vi "GetClassDependencies.vi"(0 "ClassReader in":refnum<class "ClassReader.lvclass">, 1 "DependencyVIs":T4[](array[typedef]), 2 "Attributes":T1[](array[typedef])=[{"name"="MyU8", "type"=enum."UINT8", "dimension"=0, "typeName"="", "typePath"=path "", "visibility"=enum."Protected"}, {"name"="MyStrArray", "type"=enum."STRING", "dimension"=1, "typeName"="", "typePath"=path "", "visibility"=enum."Protected"}], 5 "error in (no error)":errorcluster) -> (14 "ClassReader out":refnum<class "ClassReader.lvclass">, 15 "DependencyClassPaths":path[](array[path]), 16 "IsDependencyClassPathsAByValueClass":bool[](array[boolean]), 17 "CreateClassVIsCalled":path[](array[path]), 19 "error out":errorcluster)   [LabVIEW 2020, in "ClassReader.lvclass"]
uses:
  ClassReader.lvclass
  MethodDependencyType.ctl
  Common/ScriptingFunctions/SubVIs/Scripting_ViDependencyType.ctl
  Common/CommonVIs/CommonVIs_AttributeInfoType.ctl
  Common/CommonVIs/CommonVIs_AttributeDataType.ctl
  Common/CommonVIs/CommonVIs_VisibilityType.ctl
  ClassReader.lvclass/ClassReader.ctl
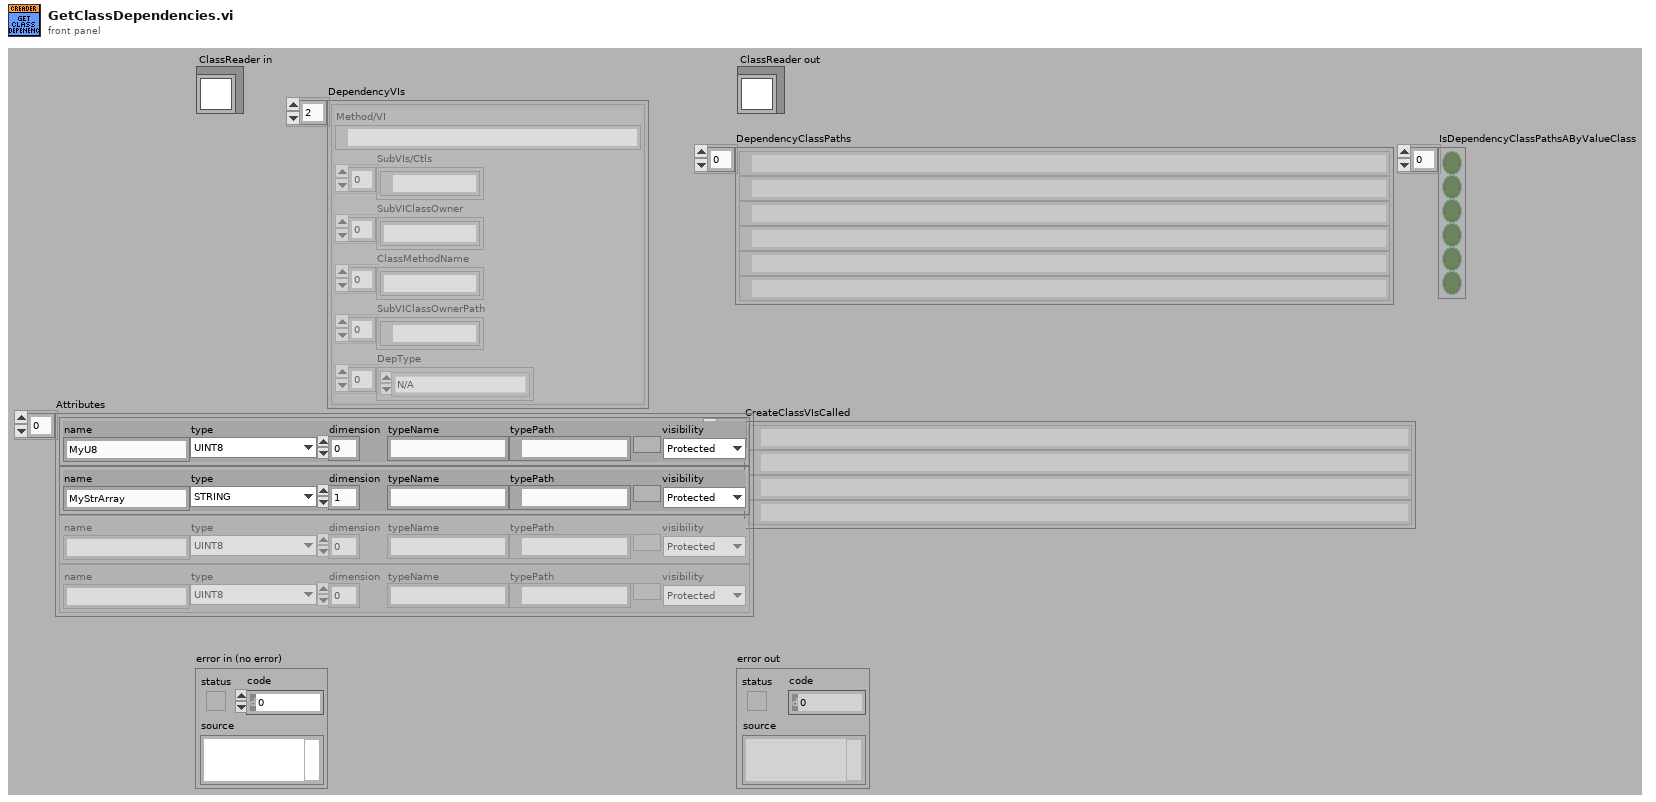
[diagram p1: front panel]
types:
  T1 = typedef "CommonVIs_AttributeInfoType.ctl" = cluster{"name":string, "type":T2, "dimension":i32, "typeName":string, "typePath":path, "visibility":T3}
  T2 = typedef "CommonVIs_AttributeDataType.ctl" = enum16{"UINT8", "INT8", "UINT16", "INT16", "UINT32", "INT32", "UINT64", "INT64", "SGL", "DBL", "EXT", "CSG", "CDB", "CXT", "TimeStamp", "STRING", "PATH", "BOOL", "ENUM", "RefNum", "VIRefNum", "LabVIEW Class", "Cluster", "Variant", "TypeDef", "Waveform", "LabVIEW Object", "Other", "void", "Set", "Map"}
  T3 = typedef "CommonVIs_VisibilityType.ctl" = enum16{"Public", "Private", "Protected"}
  T4 = typedef "ClassReader.lvclass/MethodDependencyType.ctl" = cluster{"Method/VI":path, "SubVIs/Ctls":path[], "SubVIClassOwner":string[], "ClassMethodName":string[], "SubVIClassOwnerPath":path[], "DepType":T5[]}
  T5 = typedef "Scripting_ViDependencyType.ctl" = enum16{"N/A", "Launches"}
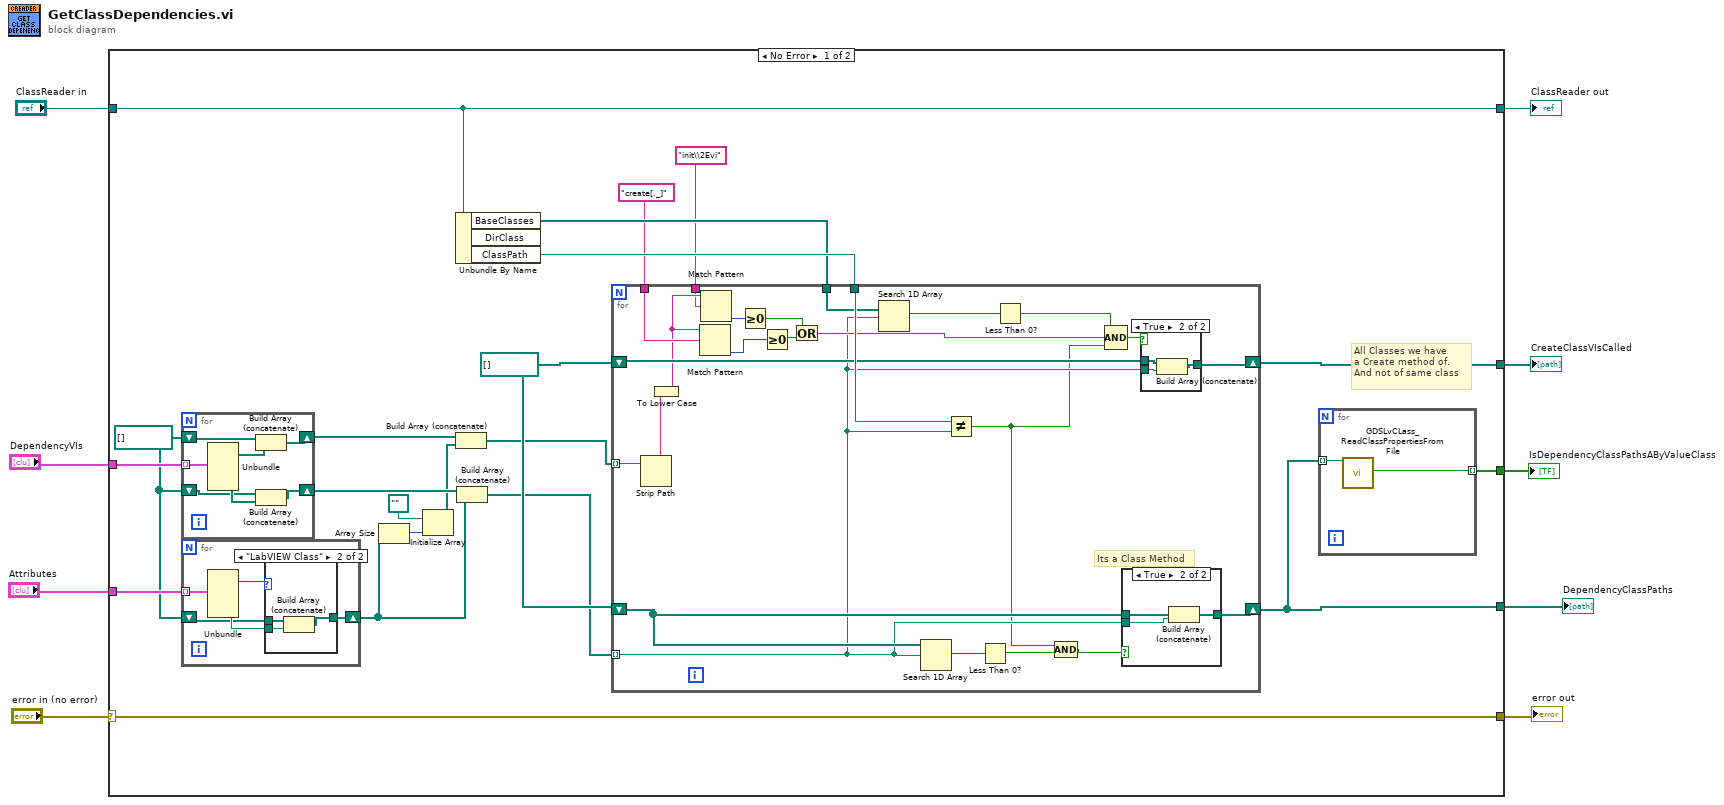
[diagram p0: block diagram]
diagram:
  n1 = case shown="No Error" "error in (no error)" {
    selector: "error in (no error)" -> [w27 w82]
    tunnel: [w27 w82] -> w8
    tunnel: [w28 w81] -> w6
    tunnel: "ClassReader in" -> [w28 w81]
    tunnel: "DependencyVIs" -> [w23 _]
    tunnel: [w10 _] -> w4
    tunnel: [w12 _] -> w3
    tunnel: "Attributes" -> [w22 _]
    tunnel: [w11 _] -> w1
    frame No Error {
      w13 = path[] []
      w29 = path[] []
      # "All Classes we have\na Create method of.\nAnd not of same class"
      n2 = for {
        tunnel: w23 -> [w80] mode=indexing
        shift-right: [w78] -> w21
        shift-left: w13 -> [w79]
        shift-right: [w75] -> w19
        shift-left: w13 -> [w74]
        n3 = Unbundle(w80) -> ("SubVIs/Ctls"=w77:path[], "SubVIClassOwnerPath"=w76:path[])  [unwired: 4 out]
        n4 = Build Array (concatenate)(w79, w77) -> (w78:path[])
        n5 = Build Array (concatenate)(w74, w76) -> (w75:path[])
      }
      n6 = for {
        tunnel: w22 -> [w69] mode=indexing
        shift-right: [w67] -> w17
        shift-left: w13 -> [w65]
        n7 = Unbundle(w69) -> ("type"=w66:T2, "typePath"=w68:path)  [unwired: 4 out]
        n8 = case shown="\"LabVIEW Class\"" w66 {
          tunnel: w65 -> [w70 w73]
          tunnel: w68 -> [_ w72]
          tunnel: [w70 w71] -> w67
          frame "UINT8", Default {
          }
          frame "LabVIEW Class" {
            n9 = Build Array (concatenate)(w73, w72) -> (w71:path[])
          }
        }
      }
      n10 = Array Size(array=w17) -> (size(s)=w16:i32)
      n11 = Initialize Array(path "" ("Path"), w16) -> (w14:path[])
      n12 = Unbundle By Name(w28) -> ("BaseClasses"=w26:path[], "ClassPath"=w30:path)  [unwired: 1 out]
      n13 = Build Array (concatenate)(w21, w14) -> (w20:path[])
      n14 = Build Array (concatenate)(w19, w17) -> (w18:path[])
      n15 = for {
        shift-right: [w54] -> w10
        shift-left: w29 -> [w55]
        tunnel: w30 -> [w53]
        shift-right: [w50] -> w12
        shift-left: w29 -> [w51]
        tunnel: w26 -> [w47]
        tunnel: w20 -> [w45] mode=indexing
        tunnel: "create[._]" ("string") -> [w43]
        tunnel: "init\\2Evi" ("string") -> [w38]
        tunnel: w18 -> [w37] mode=indexing
        # "Its a Class Method"
        n16 = Strip Path(path=w45) -> (name=w44:string)  [unwired: 1 out]
        n17 = To Lower Case(string=w44) -> (all lower case string=w42:string)
        n18 = Match Pattern(string=w42, regular expression=w43) -> (offset past match=w49:i32)  [unwired: 1 in, 3 out]
        n19 = Match Pattern(string=w42, regular expression=w38) -> (offset past match=w41:i32)  [unwired: 1 in, 3 out]
        n20 = Greater Or Equal To 0?(x=w41) -> (x >= 0?=w39:bool)
        n21 = Greater Or Equal To 0?(x=w49) -> (x >= 0?=w48:bool)
        n22 = Or(x=w39, y=w48) -> (x .or. y?=w40:bool)
        n23 = Search 1D Array(1D array=w47, element=w37) -> (index of element=w46:i32)  [unwired: 1 in]
        n24 = Search 1D Array(1D array=w55, element=w37) -> (index of element=w56:i32)  [unwired: 1 in]
        n25 = Not Equal?(x=w53, y=w37) -> (x != y?=w33:bool)
        n26 = Less Than 0?(x=w56) -> (x < 0?=w36:bool)
        n27 = Less Than 0?(x=w46) -> (x < 0?=w34:bool)
        n28 = Compound Arithmetic op=AND(w33, w36) -> (w35:bool)
        n29 = Compound Arithmetic op=AND(w34, w40, w33) -> (w52:bool)
        n30 = case shown="True" w35 {
          tunnel: w55 -> [w61 w64]
          tunnel: [w61 w63] -> w54
          tunnel: w37 -> [_ w62]
          frame False {
          }
          frame True {
            n31 = Build Array (concatenate)(w64, w62) -> (w63:path[])
          }
        }
        n32 = case shown="True" w52 {
          tunnel: w51 -> [w57 w60]
          tunnel: w37 -> [_ w59]
          tunnel: [w57 w58] -> w50
          frame False {
          }
          frame True {
            n33 = Build Array (concatenate)(w60, w59) -> (w58:path[])
          }
        }
      }
      n34 = for {
        tunnel: w10 -> [w32] mode=indexing
        tunnel: [w31] -> w11 mode=indexing
        n35 = call "GDSLvCLass_ReadClassPropertiesFromFile.vi"("LvClassPathIn"=w32) -> ("DataFlowClass"=w31:bool)  [unwired: 15 in, 3 out]
      }
    }
    frame Error {
    }
  }
  "error out" <- w8
  "ClassReader out" <- w6
  "DependencyClassPaths" <- w4
  "CreateClassVIsCalled" <- w3
  "IsDependencyClassPathsAByValueClass" <- w1
